vi "ODH_LEGO_Producer.vi"(8 "Error In":errorcluster, 9 "Time":dbl, 11 "State":T1) -> (0 "Error Out":errorcluster)   [LabVIEW 2016]
uses:
  Controls/Lego_State_Control.ctl
  Controls/Lego_ComboBox_Parameters.ctl
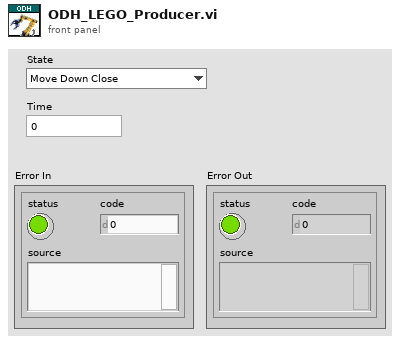
[diagram p1: front panel]
types:
  T1 = typedef "Lego_State_Control.ctl" = enum16{"Move Down Close", "Move Down Open", "Move Down Comfort Close", "Move Up Open", "Move Up Close", "Move Up Comfort Close", "Wait"}
  T2 = typedef "Lego_ComboBox_Parameters.ctl" = string
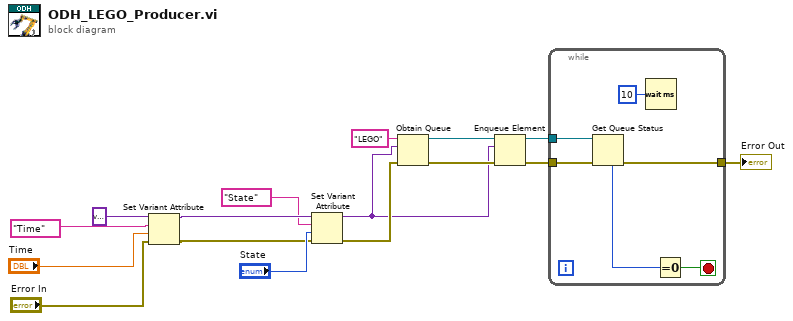
[diagram p0: block diagram]
diagram:
  n1 = Set Variant Attribute(Variant=variant, name=T2 "Time" ("Combo Box"), value="Time", error in="Error In") -> (Variant out=w11:variant, error out=w9:errorcluster)  [unwired: 1 out]
  n2 = Set Variant Attribute(Variant=w11, name=T2 "State" ("Combo Box"), value="State", error in=w9) -> (Variant out=w7:variant, error out=w8:errorcluster)  [unwired: 1 out]
  n3 = Obtain Queue(name (unnamed)="LEGO", element data type=w7, error in (no error)=w8) -> (queue out=w14:refnum<queue>, error out=w15:errorcluster)  [unwired: 2 in, 1 out]
  n4 = Enqueue Element(queue=w14, element=w7, error in (no error)=w15) -> (queue out=w2:refnum<queue>, error out=w3:errorcluster)  [unwired: 1 in, 1 out]
  n5 = while {
    tunnel: w3 -> [w22]
    tunnel: w2 -> [w21]
    tunnel: [w20] -> w1
    stop <- w18 stop-if-true
    n6 = Get Queue Status(queue=w21, error in (no error)=w22) -> (error out=w20:errorcluster, # elements in queue=w17:i32)  [unwired: 1 in, 6 out]
    n7 = Wait (ms)(milliseconds to wait=u32 10) -> ()  [unwired: 1 out]
    n8 = Equal To 0?(x=w17) -> (x = 0?=w18:bool)
  }
  "Error Out" <- w1
